vi "toggleSwitch.vi"(11 "Button":bool) -> (3 "State":bool)   [LabVIEW 2016]
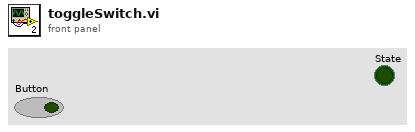
[diagram p1: front panel]
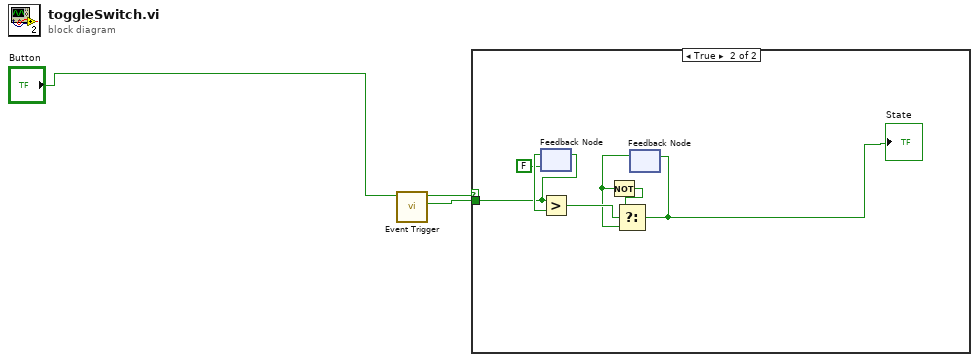
[diagram p0: block diagram]
diagram:
  n1 = call "Event Trigger.vi"("Boolean"="Button") -> ("State Passthrough"=w2:bool, "Event Trigger"=w1:bool)  [unwired: 9 in]
  n2 = case shown="True" w1 {
    tunnel: w2 -> [_ w4]
    frame False {
    }
    frame True {
      n3 = feedback #1(FALSE) -> (w10:bool)
      n4 = feedback-in #1(w4) -> ()
      n5 = Greater?(x=w4, y=w10) -> (0:w8:bool)
      n6 = feedback #2() -> (w6:bool)  [unwired: 1 in]
      n7 = Not(x=w6) -> (.not. x?=w7:bool)
      n8 = Select(t=w7, s=w8, f=w6) -> (s? t:f=w5:bool)
      "State" <- w5
      n9 = feedback-in #2(w5) -> ()
    }
  }
